vi "SignalGenerationTesting.vi"() -> ()   [LabVIEW 2013]
panel:
  in  "stop":bool
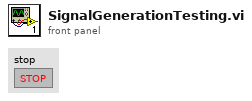
[diagram p1: front panel]
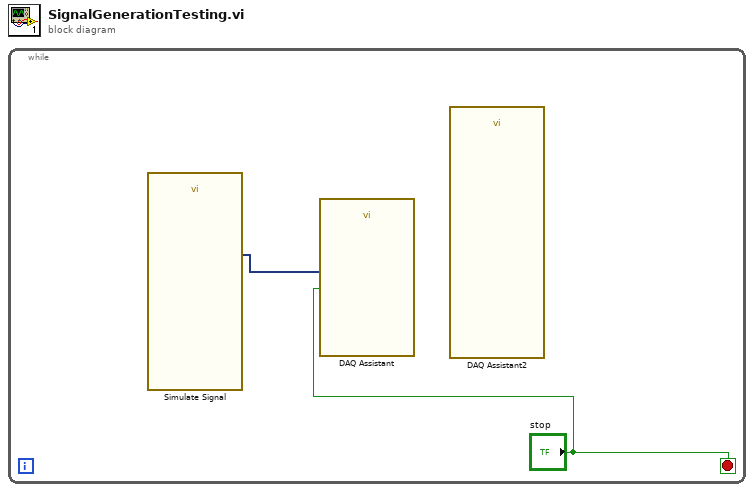
[diagram p0: block diagram]
diagram:
  n1 = while {
    stop <- "stop" stop-if-true
    n2 = call "Simulate Signal"() -> ("Sine"=w2:dynamicdata)  [unwired: 14 in, 1 out]
    n3 = call "DAQ Assistant"("data"=w2, "stop (F)"="stop") -> ()  [unwired: 15 in, 3 out]
    n4 = call "DAQ Assistant2"() -> ()  [unwired: 16 in, 4 out]
  }
